vi "Wzmacniacz_2.vi"(6 "Wartosc_poprzednia":dbl, 8 "Milisekund_na_dane":u32, 9 "Wzmocnienie":dbl, 10 "Rodzaj_wzmacniacza":T1, 11 "Sygnal_wejsciowy":dbl[](array[numeric])) -> (2 "Wartosc_poprzednia":dbl, 3 "Sygnal_wzmocniony":dbl)   [LabVIEW 2020]
doc: "VI zwraca wartosci wzmocnionego sygnalu modulujacego"
uses:
  Kontrolki/Rodzaj_wzmacniacza.ctl
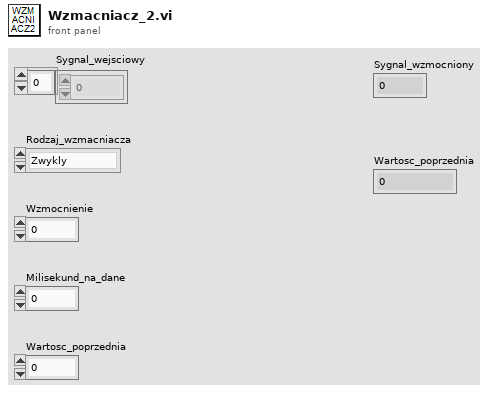
[diagram p1: front panel]
types:
  T1 = typedef "Rodzaj_wzmacniacza.ctl" = enum16{"Zwykly", "Calkujacy", "Rozniczkujacy"}
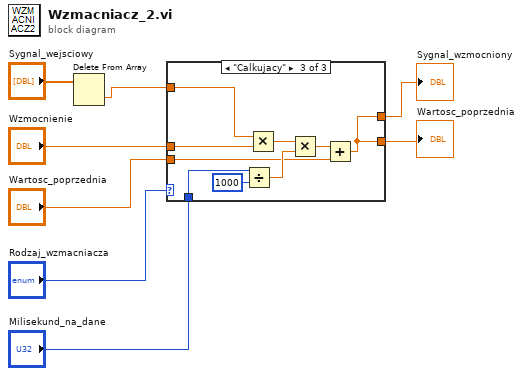
[diagram p0: block diagram]
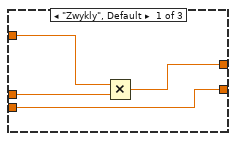
[diagram p2: hidden frame]
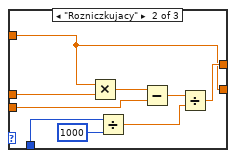
[diagram p3: hidden frame]
diagram:
  n1 = Delete From Array(array="Sygnal_wejsciowy") -> (deleted portion=w1:dbl)  [unwired: 2 in, 1 out]
  n2 = case shown="\"Calkujacy\"" "Rodzaj_wzmacniacza" {
    tunnel: w1 -> [w9 w13 w22]
    tunnel: "Wzmocnienie" -> [w12 w21 w30]
    tunnel: [w10 w13 w23] -> w5
    tunnel: "Wartosc_poprzednia" -> [w10 w20 w24]
    tunnel: [w11 w15 w23] -> w7
    tunnel: "Milisekund_na_dane" -> [_ w18 w29]
    frame "Zwykly", Default {
      n3 = Multiply(x=w9, y=w12) -> (x*y=w11:dbl)
    }
    frame "Rozniczkujacy" {
      n4 = Multiply(x=w13, y=w21) -> (x*y=w19:dbl)
      n5 = Divide(x=w18, y=1000) -> (x/y=w14:dbl)
      n6 = Subtract(x=w19, y=w20) -> (x-y=w16:dbl)
      n7 = Divide(x=w16, y=w14) -> (x/y=w15:dbl)
    }
    frame "Calkujacy" {
      n8 = Divide(x=w29, y=1000) -> (x/y=w26:dbl)
      n9 = Multiply(x=w22, y=w30) -> (x*y=w27:dbl)
      n10 = Multiply(x=w27, y=w26) -> (x*y=w25:dbl)
      n11 = Add(x=w25, y=w24) -> (x+y=w23:dbl)
    }
  }
  "Sygnal_wzmocniony" <- w7
  "Wartosc_poprzednia" <- w5
